vi "mobileyelanepaser4.vi"(6 "count hold":u64, 8 "thresh  c":dbl, 9 "thresh  b":dbl, 11 "thresh r":dbl) -> (0 "cr2":dbl=0.017, 1 "cr":dbl=1.4, 2 "cl2":dbl=0.017, 3 "cl":dbl=-1.5000000000000002)   [LabVIEW 2015]
uses:
  G_LCM.vi
  G_SEN.vi
panel:
  out "Lane_empty":dbl[](array[numeric])=[0.8601491478953653, 0.8717844136967624, 0.882947592858927, 0.8936326403234123, 0.9038337699485205, 0.9135454576426009, 0.9227624443554423, 0.9314797389261423, 0.9396926207859084, 0.9473966425143293, 0.9545876322477319, 0.9612616959383189, 0.9674152194628639, 0.9730448705798238, 0.9781476007338057, 0.9827206467064133, 0.9867615321125792, 0.9902680687415704, 0.993238357741943, 0.9956707906498045, 0.9975640502598242, 0.9989171113385246, 0.9997292411794617, 1.0, 0.9997292411794617, 0.9989171113385246, 0.9975640502598242, 0.9956707906498045, 0.993238357741943, 0.9902680687415704, 0.9867615321125792, 0.9827206467064133]
  out "blink filter":bool
  out "Lane_C_M":dbl[](array[numeric])=[0.8601491478953653, 0.8717844136967624, 0.882947592858927, 0.8936326403234123, 0.9038337699485205, 0.9135454576426009, 0.9227624443554423, 0.9314797389261423, 0.9396926207859084, 0.9473966425143293, 0.9545876322477319, 0.9612616959383189, 0.9674152194628639, 0.9730448705798238, 0.9781476007338057, 0.9827206467064133, 0.9867615321125792, 0.9902680687415704, 0.993238357741943, 0.9956707906498045, 0.9975640502598242, 0.9989171113385246, 0.9997292411794617, 1.0, 0.9997292411794617, 0.9989171113385246, 0.9975640502598242, 0.9956707906498045, 0.993238357741943, 0.9902680687415704, 0.9867615321125792, 0.9827206467064133]
  out "cr_old":dbl
  out "cl_old":dbl
  out "r_old":dbl
  out "t0":i64
  out "b_old":dbl
  out "a2":dbl
  out "b2":dbl=0.017
  out "r2":dbl
  out "dt":dbl=0.096219
  out "count":u64
  out "Lane_R_M":dbl[](array[numeric])=[0.8, 0.0036309999999999997, 0.017, 1.4]
  out "Lane_L_M":dbl[](array[numeric])=[0.8, 0.0036309999999999997, 0.017, -1.5000000000000002]
  in  "shift_c":dbl=-0.1
  in  "bias_b":dbl=0.005
  out "a":dbl=0.0036309999999999997
  out "b":dbl=0.017
  out "confidance_L":u8=2
  out "confidance_R":u8=2
  in  "bias_c":dbl=0.8
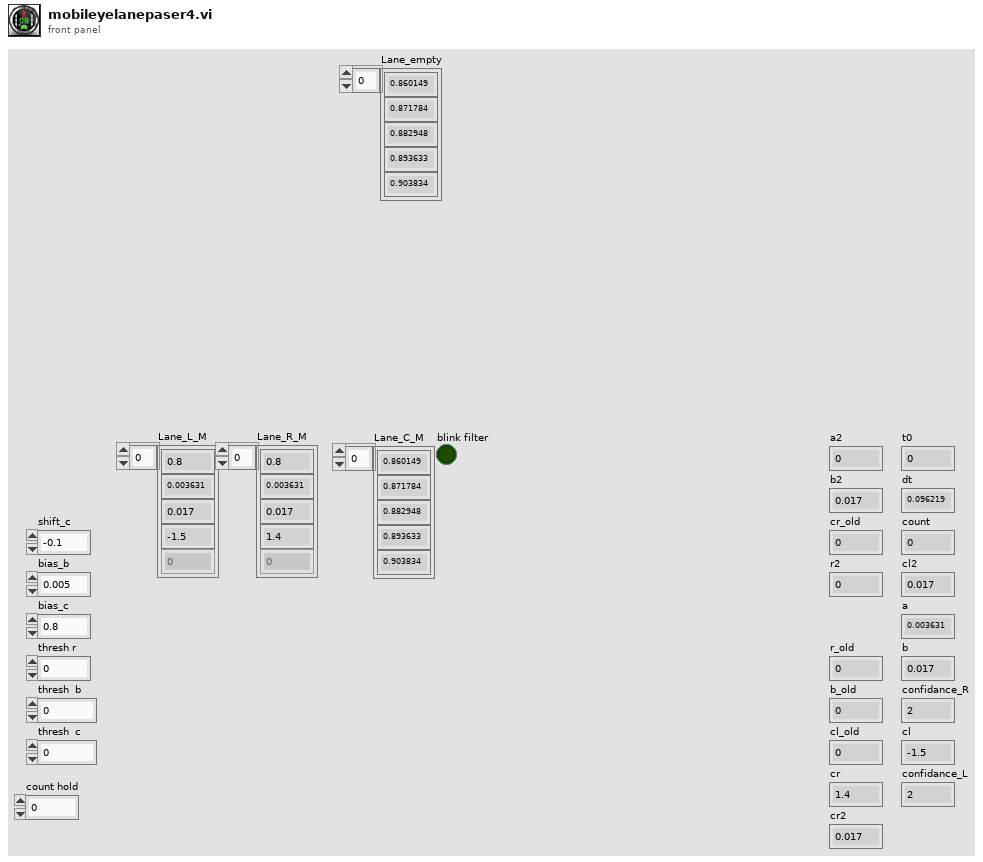
[diagram p1: front panel]
types:
  T1 = cluster{"hash":i64, "sys time":i64, "mobileye":u8[]}
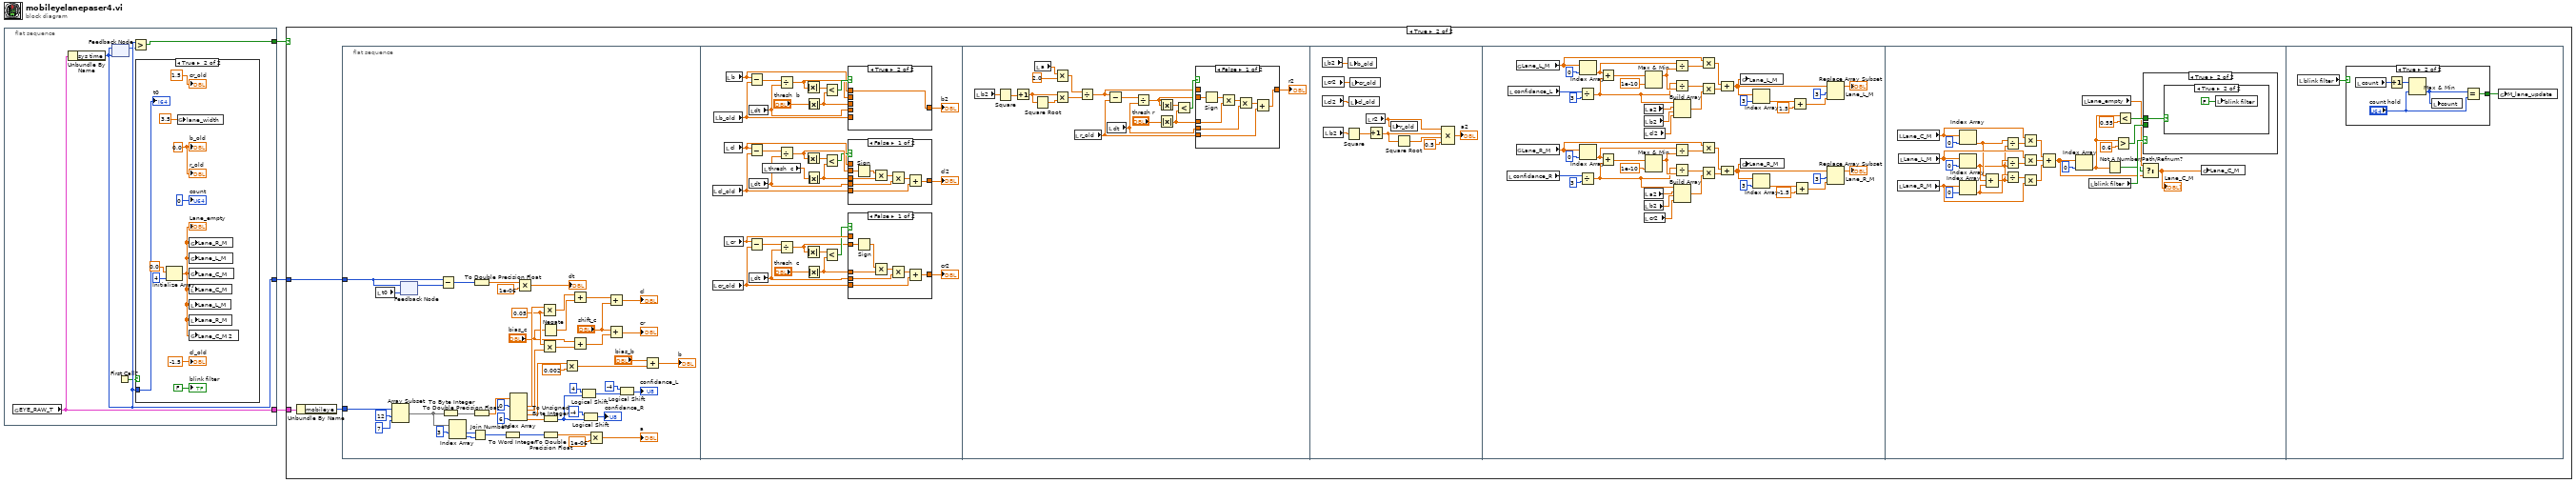
[diagram p0: block diagram]
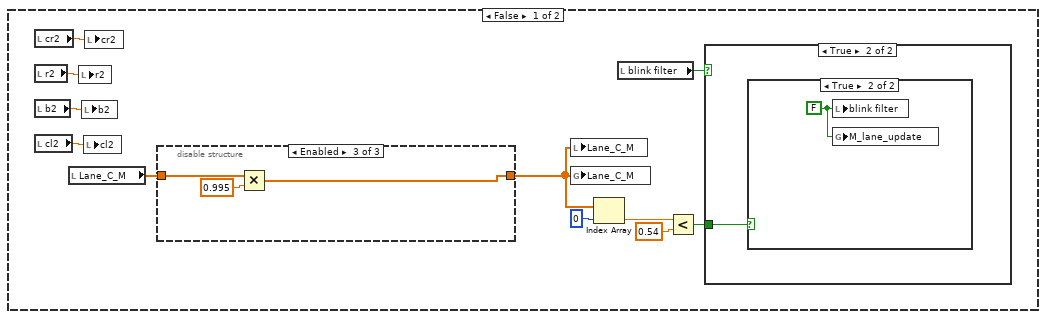
[diagram p3: hidden frame]
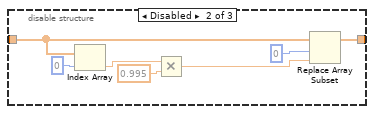
[diagram p7: hidden frame]
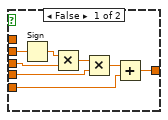
[diagram p10: hidden frame]
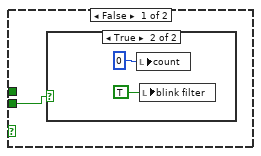
[diagram p12: hidden frame]
diagram:
  n1 = flat-sequence {
    tunnel: [w8] -> w3
    tunnel: [w7] -> w2
    tunnel: [w6] -> w1
    frame #0 {
      n2 = global read "G_LCM.vi" "EYE_RAW_T"() -> (w8:T1)
      n3 = Unbundle By Name(w8) -> ("sys time"=w6:i64)
      n4 = feedback #1(w6) -> (w4:i64)
      n5 = feedback-in #1(w6) -> ()
      n6 = First Call?() -> (First Call?: T/F=w5:bool)
      n7 = Greater?(x=w6, y=w4) -> (0:w7:bool)
      n8 = case shown="True" w5 {
        tunnel: w6 -> [_ w14]
        frame False {
        }
        frame True {
          w13 = 0.0 ("dt2")
          n9 = Initialize Array(0.0 ("element"), 4 ("dimension size")) -> (w9:dbl[])
          "Lane_empty" <- w9
          n10 = global write "G_SEN.vi" "lane_width"(3.5 ("lane_width")) -> ()
          n11 = global write "G_SEN.vi" "Lane_R_M"(w9) -> ()
          n12 = global write "G_SEN.vi" "Lane_L_M"(w9) -> ()
          n13 = global write "G_SEN.vi" "Lane_C_M"(w9) -> ()
          n14 = local write "Lane_C_M"(w9) -> ()
          n15 = local write "Lane_L_M"(w9) -> ()
          n16 = local write "Lane_R_M"(w9) -> ()
          n17 = global write "G_SEN.vi" "Lane_C_M 2"(w9) -> ()
          "count" <- u64 0
          "b_old" <- w13
          "t0" <- w14
          "r_old" <- w13
          "cl_old" <- -1.5 ("cl_old")
          "cr_old" <- 1.5 ("cr_old")
          "blink filter" <- FALSE
        }
      }
    }
  }
  n18 = case shown="True" w2 {
    tunnel: w3 -> [_ w44]
    tunnel: w1 -> [_ w43]
    frame False {
      n19 = local read "cr2"() -> (w27:dbl)
      n20 = local read "r2"() -> (w29:dbl)
      n21 = local read "b2"() -> (w28:dbl)
      n22 = local read "cl2"() -> (w26:dbl)
      n23 = local read "Lane_C_M"() -> (w25:dbl[])
      n24 = local write "r2"(w29) -> ()
      n25 = local write "b2"(w28) -> ()
      n26 = local write "cl2"(w26) -> ()
      n27 = local write "cr2"(w27) -> ()
      n28 = disable-structure shown="Enabled" {
        disable-tunnel: w25 -> [w32 w34 w41]
        disable-tunnel: [w32 w33 w40] -> w20
        frame Disabled {
        }
        frame Disabled {
          n29 = Index Array(array=w34, index=0) -> (element=w37:dbl)
          n30 = Multiply(x=w37, y=0.995) -> (x*y=w35:dbl)
          n31 = Replace Array Subset(array=w34, new element=w35, index=0) -> (w33:dbl[])
        }
        frame Enabled {
          n32 = Multiply(x=w41, y=0.995) -> (x*y=w40:dbl[])
        }
      }
      n33 = local write "Lane_C_M"(w20) -> ()
      n34 = global write "G_SEN.vi" "Lane_C_M"(w20) -> ()
      n35 = Index Array(array=w20, index=0) -> (element=w19:dbl)
      n36 = local read "blink filter"() -> (w24:bool)
      n37 = Less?(x=w19, y=0.54) -> (x < y?=w22:bool)
      n38 = case shown="True" w24 {
        tunnel: w22 -> [_ w30]
        frame False {
        }
        frame True {
          n39 = case shown="True" w30 {
            frame False {
            }
            frame True {
              w31 = FALSE ("blink filter")
              n40 = local write "blink filter"(w31) -> ()
              n41 = global write "G_SEN.vi" "M_lane_update"(w31) -> ()
            }
          }
        }
      }
    }
    frame True {
      n42 = Unbundle By Name(w44) -> ("mobileye"=w45:u8[])
      n43 = flat-sequence {
        tunnel: w45 -> [w71]
        tunnel: w43 -> [w58]
        frame #0 {
          w55 = 0.05 ("y")
          n44 = local read "t0"() -> (w57:i64)
          n45 = Array Subset(array=w71, index=12, length=7) -> (w70:u8[])
          n46 = feedback #2(w57) -> (w59:i64)
          n47 = feedback-in #2(w58) -> ()
          n48 = Subtract(x=w58, y=w59) -> (x-y=w60:i64)
          n49 = To Byte Integer(number=w70) -> (8bit integer=w90:i8[])
          n50 = Index Array(array=w70, index #1=3 ("index")) -> (element #1=w84:u8, element #2=w83:u8)  [unwired: 1 in]
          n51 = Join Numbers(hi=w84, lo=w83) -> ((hi.lo)=w82:u16)
          n52 = To Double Precision Float(number=w60) -> (double precision float=w63:dbl)
          n53 = To Double Precision Float(number=w90) -> (double precision float=w89:dbl[])
          n54 = To Word Integer(number=w82) -> (16bit integer=w81:i16)
          n55 = Index Array(array=w89, index #1=0 ("index"), index #4=6 ("index")) -> (element #1=w88:dbl, element #2=w87:dbl, element #3=w86:dbl, element #4=w77:dbl)  [unwired: 2 in]
          n56 = Multiply(x=w63, y=1e-06) -> (x*y=→"dt":dbl)
          n57 = Multiply(x=w88, y=w55) -> (x*y=w53:dbl)
          n58 = Multiply(x=w55, y=w87) -> (x*y=w54:dbl)
          n59 = Negate(x="bias_c") -> (-x=w51:dbl)
          n60 = To Unsigned Byte Integer(number=w77) -> (unsigned 8bit integer=w75:u8)
          n61 = To Double Precision Float(number=w81) -> (double precision float=w64:dbl)
          n62 = Multiply(x=w86, y=0.002) -> (x*y=w67:dbl)
          n63 = Add(x=w53, y=w51) -> (x+y=w50:dbl)
          n64 = Add(x="bias_c", y=w54) -> (x+y=w48:dbl)
          n65 = Logical Shift(y=i16 4, x=w75) -> (x << y=w73:u8)
          n66 = Logical Shift(y=i16 -4, x=w75) -> (x << y=→"confidance_R":u8)
          n67 = Multiply(x=w64, y=1e-06) -> (x*y=→"a":dbl)
          n68 = Add(x=w50, y="shift_c") -> (x+y=→"cl":dbl)
          n69 = Add(x="shift_c", y=w48) -> (x+y=→"cr":dbl)
          n70 = Logical Shift(y=i16 -4, x=w73) -> (x << y=→"confidance_L":u8)
          n71 = Add(x="bias_b", y=w67) -> (x+y=→"b":dbl)
        }
        frame #1 {
          n72 = local read "cl_old"() -> (w114:dbl)
          n73 = local read "cr_old"() -> (w95:dbl)
          n74 = local read "b_old"() -> (w115:dbl)
          n75 = local read "cl"() -> (w106:dbl)
          n76 = local read "cr"() -> (w104:dbl)
          n77 = local read "b"() -> (w105:dbl)
          n78 = Subtract(x=w105, y=w115) -> (x-y=w122:dbl)
          n79 = Subtract(x=w106, y=w114) -> (x-y=w108:dbl)
          n80 = Subtract(x=w104, y=w95) -> (x-y=w102:dbl)
          n81 = local read "dt"() -> (w116:dbl)
          n82 = local read "dt"() -> (w113:dbl)
          n83 = local read "dt"() -> (w96:dbl)
          n84 = local read "thresh  c"() -> (w94:dbl)
          n85 = Divide(x=w122, y=w116) -> (x/y=w118:dbl)
          n86 = Divide(x=w108, y=w113) -> (x/y=w111:dbl)
          n87 = Divide(x=w102, y=w96) -> (x/y=w98:dbl)
          n88 = Absolute Value(x=w118) -> (abs(x)=w121:dbl)
          n89 = Absolute Value(x=w111) -> (abs(x)=w109:dbl)
          n90 = Absolute Value(x=w98) -> (abs(x)=w101:dbl)
          n91 = Absolute Value(x="thresh  b") -> (abs(x)=w117:dbl)
          n92 = Absolute Value(x=w94) -> (abs(x)=w112:dbl)
          n93 = Absolute Value(x="thresh  c") -> (abs(x)=w97:dbl)
          n94 = Less?(x=w121, y=w117) -> (x < y?=w120:bool)
          n95 = Less?(x=w109, y=w112) -> (x < y?=w110:bool)
          n96 = Less?(x=w101, y=w97) -> (x < y?=w100:bool)
          n97 = case shown="True" w120 {
            tunnel: [w148 w150] -> w123
            tunnel: w118 -> [w146 _]
            tunnel: w117 -> [w145 _]
            tunnel: w116 -> [w143 _]
            tunnel: w115 -> [w142 _]
            tunnel: w105 -> [_ w150]
            frame False {
              n98 = Sign(1:w146) -> (0:w144:dbl)
              n99 = Multiply(x=w144, y=w145) -> (x*y=w149:dbl)
              n100 = Multiply(x=w149, y=w143) -> (x*y=w147:dbl)
              n101 = Add(x=w147, y=w142) -> (x+y=w148:dbl)
            }
            frame True {
            }
          }
          "b2" <- w123
          n102 = case shown="False" w110 {
            tunnel: [w139 w141] -> w107
            tunnel: w111 -> [w137 _]
            tunnel: w112 -> [w136 _]
            tunnel: w113 -> [w134 _]
            tunnel: w114 -> [w133 _]
            tunnel: w106 -> [_ w141]
            frame False {
              n103 = Sign(1:w137) -> (0:w135:dbl)
              n104 = Multiply(x=w135, y=w136) -> (x*y=w140:dbl)
              n105 = Multiply(x=w140, y=w134) -> (x*y=w138:dbl)
              n106 = Add(x=w138, y=w133) -> (x+y=w139:dbl)
            }
            frame True {
            }
          }
          "cl2" <- w107
          n107 = case shown="False" w100 {
            tunnel: [w130 w132] -> w103
            tunnel: w98 -> [w128 _]
            tunnel: w97 -> [w127 _]
            tunnel: w96 -> [w125 _]
            tunnel: w95 -> [w124 _]
            tunnel: w104 -> [_ w132]
            frame False {
              n108 = Sign(1:w128) -> (0:w126:dbl)
              n109 = Multiply(x=w126, y=w127) -> (x*y=w131:dbl)
              n110 = Multiply(x=w131, y=w125) -> (x*y=w129:dbl)
              n111 = Add(x=w129, y=w124) -> (x+y=w130:dbl)
            }
            frame True {
            }
          }
          "cr2" <- w103
        }
        frame #2 {
          n112 = local read "b2"() -> (w156:dbl)
          n113 = Square(x=w156) -> (x^2=w157:dbl)
          n114 = Increment(x=w157) -> (x+1=w159:dbl)
          n115 = Square Root(x=w159) -> (sqrt(x)=w158:dbl)
          n116 = local read "a"() -> (w153:dbl)
          n117 = Multiply(x=w153, y=2.0) -> (x*y=w155:dbl)
          n118 = Multiply(x=w159, y=w158) -> (x*y=w160:dbl)
          n119 = local read "r_old"() -> (w151:dbl)
          n120 = Divide(x=w155, y=w160) -> (x/y=w161:dbl)
          n121 = Subtract(x=w161, y=w151) -> (x-y=w168:dbl)
          n122 = local read "dt"() -> (w152:dbl)
          n123 = Divide(x=w168, y=w152) -> (x/y=w163:dbl)
          n124 = Absolute Value(x=w163) -> (abs(x)=w167:dbl)
          n125 = Absolute Value(x="thresh r") -> (abs(x)=w162:dbl)
          n126 = Less?(x=w167, y=w162) -> (x < y?=w166:bool)
          n127 = case shown="False" w166 {
            tunnel: [w175 w177] -> w165
            tunnel: w163 -> [w173 _]
            tunnel: w162 -> [w172 _]
            tunnel: w152 -> [w170 _]
            tunnel: w161 -> [_ w177]
            tunnel: w151 -> [w169 _]
            frame False {
              n128 = Sign(1:w173) -> (0:w171:dbl)
              n129 = Multiply(x=w171, y=w172) -> (x*y=w176:dbl)
              n130 = Multiply(x=w176, y=w170) -> (x*y=w174:dbl)
              n131 = Add(x=w174, y=w169) -> (x+y=w175:dbl)
            }
            frame True {
            }
          }
          "r2" <- w165
        }
        frame #3 {
          n132 = local read "b2"() -> (w181:dbl)
          n133 = local read "cr2"() -> (w178:dbl)
          n134 = local read "cl2"() -> (w179:dbl)
          n135 = local read "b2"() -> (w187:dbl)
          n136 = Square(x=w187) -> (x^2=w186:dbl)
          n137 = local write "b_old"(w181) -> ()
          n138 = local write "cl_old"(w179) -> ()
          n139 = local write "cr_old"(w178) -> ()
          n140 = local read "r2"() -> (w180:dbl)
          n141 = Increment(x=w186) -> (x+1=w184:dbl)
          n142 = local write "r_old"(w180) -> ()
          n143 = Square Root(x=w184) -> (sqrt(x)=w185:dbl)
          n144 = Compound Arithmetic op=MULTIPLY(w180, w184, w185, 0.5 ("value")) -> (→"a2":dbl)
        }
        frame #4 {
          n145 = local read "confidance_R"() -> (w189:u8)
          n146 = local read "confidance_L"() -> (w188:u8)
          n147 = global read "G_SEN.vi" "Lane_L_M"() -> (w197:dbl[])
          n148 = global read "G_SEN.vi" "Lane_R_M"() -> (w231:dbl[])
          n149 = Index Array(array=w197, index=0) -> (element=w195:dbl)
          n150 = Divide(x=w188, y=u8 3) -> (x/y=w191:dbl)
          n151 = Index Array(array=w231, index=0) -> (element=w233:dbl)
          n152 = Divide(x=w189, y=u8 3) -> (x/y=w192:dbl)
          n153 = Add(x=w195, y=w191) -> (x+y=w206:dbl)
          n154 = Add(x=w233, y=w192) -> (x+y=w222:dbl)
          n155 = local read "a2"() -> (w199:dbl)
          n156 = local read "b2"() -> (w200:dbl)
          n157 = local read "cl2"() -> (w201:dbl)
          n158 = local read "a2"() -> (w229:dbl)
          n159 = local read "b2"() -> (w228:dbl)
          n160 = local read "cr2"() -> (w227:dbl)
          n161 = Max & Min(x=w206, y=1e-10) -> (max(x,y)=w207:dbl)  [unwired: 1 out]
          n162 = Max & Min(x=w222, y=1e-10) -> (max(x,y)=w221:dbl)  [unwired: 1 out]
          n163 = Divide(x=w195, y=w207) -> (x/y=w196:dbl)
          n164 = Divide(x=w191, y=w207) -> (x/y=w202:dbl)
          n165 = Build Array(w191, w199, w200, w201) -> (w203:dbl[])
          n166 = Divide(x=w233, y=w221) -> (x/y=w232:dbl)
          n167 = Divide(x=w192, y=w221) -> (x/y=w226:dbl)
          n168 = Build Array(w192, w229, w228, w227) -> (w225:dbl[])
          n169 = Multiply(x=w197, y=w196) -> (x*y=w198:dbl[])
          n170 = Multiply(x=w202, y=w203) -> (x*y=w204:dbl[])
          n171 = Multiply(x=w231, y=w232) -> (x*y=w230:dbl[])
          n172 = Multiply(x=w226, y=w225) -> (x*y=w224:dbl[])
          n173 = Compound Arithmetic op=ADD(w198, w204) -> (w211:dbl[])
          n174 = Compound Arithmetic op=ADD(w230, w224) -> (w217:dbl[])
          n175 = global write "G_SEN.vi" "Lane_L_M"(w211) -> ()
          n176 = global write "G_SEN.vi" "Lane_R_M"(w217) -> ()
          n177 = Index Array(array=w211, index=3) -> (element=w209:dbl)
          n178 = Index Array(array=w217, index=3) -> (element=w219:dbl)
          n179 = Add(x=w209, y=1.5) -> (x+y=w213:dbl)
          n180 = Add(x=w219, y=-1.5) -> (x+y=w215:dbl)
          n181 = Replace Array Subset(array=w211, new element=w213, index=3) -> (→"Lane_L_M":dbl[])
          n182 = Replace Array Subset(array=w217, new element=w215, index=3) -> (→"Lane_R_M":dbl[])
        }
        frame #5 {
          n183 = local read "Lane_C_M"() -> (w249:dbl[])
          n184 = local read "Lane_R_M"() -> (w248:dbl[])
          n185 = local read "Lane_L_M"() -> (w254:dbl[])
          n186 = Index Array(array=w249, index=0) -> (element=w253:dbl)
          n187 = Index Array(array=w254, index=0) -> (element=w252:dbl)
          n188 = Index Array(array=w248, index=0) -> (element=w251:dbl)
          n189 = Compound Arithmetic op=ADD(w253, w252, w251) -> (w250:dbl)
          n190 = Divide(x=w253, y=w250) -> (x/y=w261:dbl)
          n191 = Divide(x=w252, y=w250) -> (x/y=w259:dbl)
          n192 = Divide(x=w251, y=w250) -> (x/y=w247:dbl)
          n193 = Multiply(x=w249, y=w261) -> (x*y=w260:dbl[])
          n194 = Multiply(x=w254, y=w259) -> (x*y=w257:dbl[])
          n195 = Multiply(x=w247, y=w248) -> (x*y=w255:dbl[])
          n196 = Compound Arithmetic op=ADD(w260, w257, w255) -> (w238:dbl[])
          n197 = Index Array(array=w238, index=0) -> (element=w240:dbl)
          n198 = local read "Lane_empty"() -> (w237:dbl[])
          n199 = local read "blink filter"() -> (w245:bool)
          n200 = Not A Number/Path/Refnum?(number/path/refnum=w240) -> (NaN/Path/Refnum?=w239:bool)
          n201 = Greater?(x=w240, y=0.6) -> (0:w244:bool)
          n202 = Less?(x=w240, y=0.55) -> (x < y?=w241:bool)
          n203 = Select(t=w237, s=w239, f=w238) -> (s? t:f=w236:dbl[])
          "Lane_C_M" <- w236
          n204 = case shown="True" w245 {
            tunnel: w244 -> [w263 _]
            tunnel: w241 -> [_ w266]
            frame False {
              n205 = case shown="True" w263 {
                frame False {
                }
                frame True {
                  n206 = local write "count"(u64 0 ("count")) -> ()
                  n207 = local write "blink filter"(TRUE ("blink filter")) -> ()
                }
              }
            }
            frame True {
              n208 = case shown="True" w266 {
                frame False {
                }
                frame True {
                  n209 = local write "blink filter"(FALSE ("blink filter")) -> ()
                }
              }
            }
          }
          n210 = global write "G_SEN.vi" "Lane_C_M"(w236) -> ()
        }
        frame #6 {
          n211 = local read "blink filter"() -> (w269:bool)
          n212 = case shown="True" w269 {
            tunnel: [_ w270] -> w268
            frame False {
            }
            frame True {
              n213 = local read "count"() -> (w274:u64)
              n214 = Increment(x=w274) -> (x+1=w273:u64)
              n215 = Max & Min(x=w273, y="count hold") -> (min(x,y)=w272:u64)  [unwired: 1 out]
              n216 = local write "count"(w272) -> ()
              n217 = Equal?(x=w272, y="count hold") -> (x = y?=w270:bool)
            }
          }
          n218 = global write "G_SEN.vi" "M_lane_update"(w268) -> ()
        }
      }
    }
  }
